vi "sequence.vi"(10 "input":T2(array[cluster]) {"hold" format="%#_6p"; "distance" format="%#_6p"; "final vel." format="%#_6p"}, 11 "initial vel.":dbl format="%#_6p") -> (0 "total t":dbl caption="total time (s)", 1 "max a":dbl caption="max a (m /s^2)", 2 "stages":T1[](array[typedef]) {"t (s)" format="%#_6e"; "v_i (m/s)" format="%#_6e"; "a (m / s^2)" format="%#_6e"; "d (m)" format="%#_6e"; "v_f (m/s)" format="%#_6e"}, 3 "valid":bool, 4 "total d":dbl caption="total distance (m)")   [LabVIEW 2017, in "wf.lvlib" / "wf_tools.lvlib"]
uses:
  wf_tools.lvlib
  stage.ctl
panel:
  in  "stage":T1 {"t (s)" format="%#_6e"; "v_i (m/s)" format="%#_6e"; "a (m / s^2)" format="%#_6e"; "d (m)" format="%#_6e"; "v_f (m/s)" format="%#_6e"}
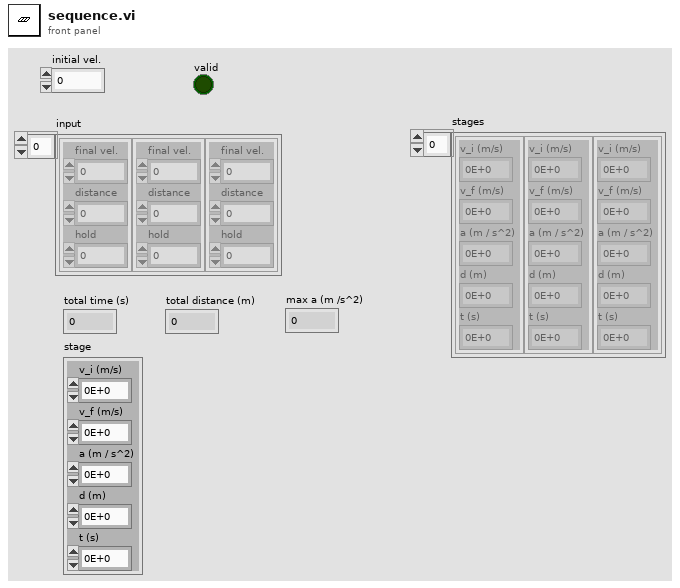
[diagram p1: front panel]
types:
  T1 = typedef "wf.lvlib/wf_tools.lvlib/stage.ctl" = cluster{"v_i (m/s)":dbl, "v_f (m/s)":dbl, "a (m / s^2)":dbl, "d (m)":dbl, "t (s)":dbl}
  T2 = cluster{"final vel.":dbl, "distance":dbl, "hold":dbl}[]
  T3 = cluster{"u (m/s)":dbl, "v (m/s)":dbl, "a (m / s^2)":dbl, "s (m)":dbl, "t (s)":dbl}[]
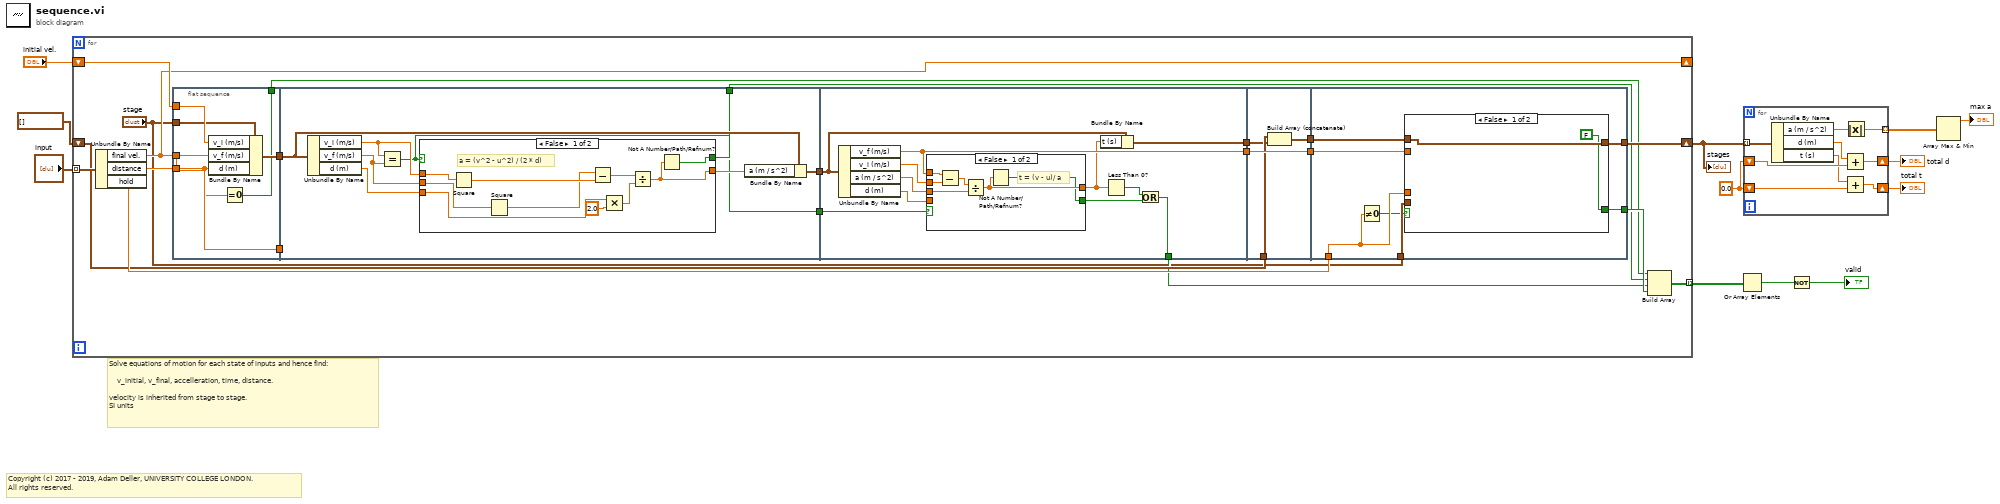
[diagram p0: block diagram]
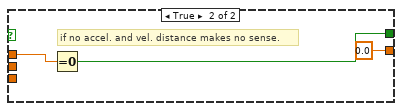
[diagram p2: hidden frame]
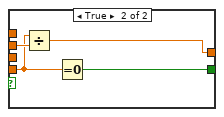
[diagram p3: hidden frame]
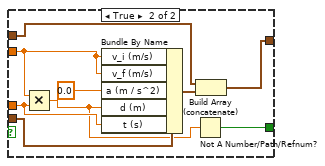
[diagram p4: hidden frame]
diagram:
  w3 = 0.0 ("s (m)")
  # "Copyright (c) 2017 - 2019, Adam Deller, UNIVERSITY COLLEGE LONDON.\nAll rights reserved."
  # "Solve equations of motion for each state of inputs and hence find:\n\n    v_initial, v_final, accelleration, time, distance. \n\nvelocity is inherited from stage to stage.\nSI units"
  n1 = for {
    tunnel: "input" -> [w33] mode=indexing
    shift-right: [w30] -> _
    shift-left: "initial vel." -> [w32]
    shift-right: [w20] -> w6
    shift-left: T3 [] ("stages 2") -> [w23]
    tunnel: [w17] -> w9 mode=indexing
    n2 = Unbundle By Name(w33) -> ("final vel."=w30:dbl, "distance"=w31:dbl, "hold"=w26:dbl)
    n3 = flat-sequence {
      tunnel: w32 -> [w39]
      tunnel: w31 -> [w35]
      tunnel: w30 -> [w36]
      tunnel: [w38] -> w29
      tunnel: "stage" -> [w37]
      tunnel: [w36] -> w27
      tunnel: [w34] -> w16
      tunnel: w29 -> [w46]
      tunnel: [w45] -> w28
      tunnel: w27 -> [_]
      tunnel: [w41] -> w15
      tunnel: [w40] -> w14
      tunnel: w28 -> [w69]
      tunnel: [w68] -> w25
      tunnel: [w67] -> w22
      tunnel: [w61] -> w18
      tunnel: w14 -> [w66]
      tunnel: w25 -> [w85]
      tunnel: [w85] -> w24
      tunnel: w23 -> [w84]
      tunnel: w22 -> [w83]
      tunnel: [w82] -> w21
      tunnel: "stage" -> [w92]
      tunnel: w24 -> [w91]
      tunnel: w26 -> [w87]
      tunnel: w21 -> [w90]
      tunnel: [w89] -> w20
      tunnel: [w88] -> w19
      frame #0 {
        n4 = Bundle By Name(cluster=w37, "v_i (m/s)"=w39, "v_f (m/s)"=w36, "d (m)"=w35) -> (w38:T1)
        n5 = Equal To 0?(x=w35) -> (x = 0?=w34:bool)
      }
      frame #1 {
        n6 = Unbundle By Name(w46) -> ("v_i (m/s)"=w43:dbl, "v_f (m/s)"=w42:dbl, "d (m)"=w47:dbl)
        n7 = Equal?(x=w43, y=w42) -> (x = y?=w40:bool)
        n8 = case shown="False" w40 {
          tunnel: w42 -> [w53 _]
          tunnel: w43 -> [w52 w59]
          tunnel: w47 -> [w50 _]
          tunnel: [w49 0.0] -> w44
          tunnel: [w48 w58] -> w41
          frame False {
            # "a = (v^2 - u^2) / (2 * d)"
            n9 = Square(x=w52) -> (x^2=w57:dbl)
            n10 = Square(x=w53) -> (x^2=w56:dbl)
            n11 = Subtract(x=w56, y=w57) -> (x-y=w55:dbl)
            n12 = Multiply(x=w50, y=2.0) -> (x*y=w54:dbl)
            n13 = Divide(x=w55, y=w54) -> (x/y=w49:dbl)
            n14 = Not A Number/Path/Refnum?(number/path/refnum=w49) -> (NaN/Path/Refnum?=w48:bool)
          }
          frame True {
            # "if no accel. and vel. distance makes no sense."
            n15 = Equal To 0?(x=w59) -> (x = 0?=w58:bool)
          }
        }
        n16 = Bundle By Name(cluster=w46, "a (m / s^2)"=w44) -> (w45:T1)
      }
      frame #2 {
        n17 = Unbundle By Name(w69) -> ("v_f (m/s)"=w68:dbl, "v_i (m/s)"=w71:dbl, "a (m / s^2)"=w70:dbl, "d (m)"=w65:dbl)
        n18 = case shown="False" w66 {
          tunnel: w71 -> [w77 w81]
          tunnel: w70 -> [w75 _]
          tunnel: w68 -> [w74 _]
          tunnel: [w73 w80] -> w64
          tunnel: [w72 w78] -> w62
          tunnel: w65 -> [_ w79]
          frame False {
            # "t = (v - u)/ a"
            n19 = Subtract(x=w74, y=w77) -> (x-y=w76:dbl)
            n20 = Divide(x=w76, y=w75) -> (x/y=w73:dbl)
            n21 = Not A Number/Path/Refnum?(number/path/refnum=w73) -> (NaN/Path/Refnum?=w72:bool)
          }
          frame True {
            n22 = Divide(x=w79, y=w81) -> (x/y=w80:dbl)
            n23 = Equal To 0?(x=w79) -> (x = 0?=w78:bool)
          }
        }
        n24 = Bundle By Name(cluster=w69, "t (s)"=w64) -> (w67:T1)
        n25 = Less Than 0?(x=w64) -> (x < 0?=w63:bool)
        n26 = Or(x=w63, y=w62) -> (x .or. y?=w61:bool)
      }
      frame #3 {
        n27 = Build Array (concatenate)(w84, w83) -> (w82:T1[])
      }
      frame #4 {
        n28 = Not Equal To 0?(x=w87) -> (x != 0?=w86:bool)
        n29 = case shown="False" w86 {
          tunnel: w92 -> [_ w98]
          tunnel: w91 -> [_ w102]
          tunnel: w87 -> [_ w101]
          tunnel: w90 -> [w94 w100]
          tunnel: [w94 w97] -> w89
          tunnel: [FALSE w95] -> w88
          frame False {
          }
          frame True {
            n30 = Multiply(x=w102, y=w101) -> (x*y=w96:dbl)
            n31 = Bundle By Name(cluster=w98, "v_i (m/s)"=w102, "v_f (m/s)"=w102, "a (m / s^2)"=0.0 ("a"), "d (m)"=w96, "t (s)"=w101) -> (w99:T1)
            n32 = Not A Number/Path/Refnum?(number/path/refnum=w96) -> (NaN/Path/Refnum?=w95:bool)
            n33 = Build Array (concatenate)(w100, w99) -> (w97:T1[])
          }
        }
      }
    }
    n34 = Build Array(w16, w15, w18, w19) -> (w17:bool[])
  }
  "stages" <- w6
  n35 = Or Array Elements(Boolean array=w9) -> (logical OR=w8:bool)
  n36 = for {
    tunnel: w6 -> [w112] mode=indexing
    tunnel: [w104] -> w5 mode=indexing
    shift-right: [w109] -> w2
    shift-left: w3 -> [w111]
    shift-right: [w106] -> w1
    shift-left: w3 -> [w108]
    n37 = Unbundle By Name(w112) -> ("a (m / s^2)"=w105:dbl, "d (m)"=w110:dbl, "t (s)"=w107:dbl)
    n38 = Add(x=w110, y=w111) -> (x+y=w109:dbl)
    n39 = Add(x=w107, y=w108) -> (x+y=w106:dbl)
    n40 = Absolute Value(x=w105) -> (abs(x)=w104:dbl)
  }
  "total d" <- w2
  "total t" <- w1
  n41 = Not(x=w8) -> (.not. x?=→"valid":bool)
  n42 = Array Max & Min(array=w5) -> (max value=→"max a":dbl)  [unwired: 3 out]
